vi "Setup.vi"(8 "error in (no error)":errorcluster, 10 "Setup Setting":T1 {"Interface:CAN:Termination" items=["Off", "On"]}, 11 "PXI 8513 in":refnum<class "PXI 8513.lvclass">) -> (0 "error out":errorcluster, 3 "PXI 8513 out":refnum<class "PXI 8513.lvclass">)   [LabVIEW 2023, in "CAN.lvlib" / "PXI 8513.lvclass"]
uses:
  PXI 8513.lvclass
  PXI 8513.lvclass/PXI 8513.ctl
  <resource>/objmgr/xnet.rc
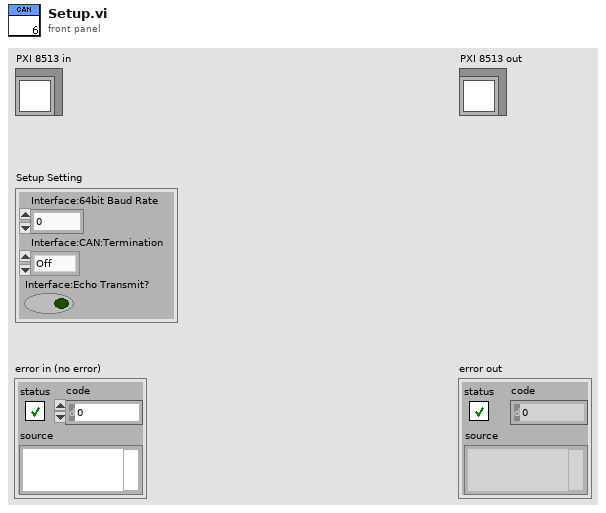
[diagram p1: front panel]
types:
  T1 = cluster{"Interface:64bit Baud Rate":u64, "Interface:CAN:Termination":u32, "Interface:Echo Transmit?":bool}
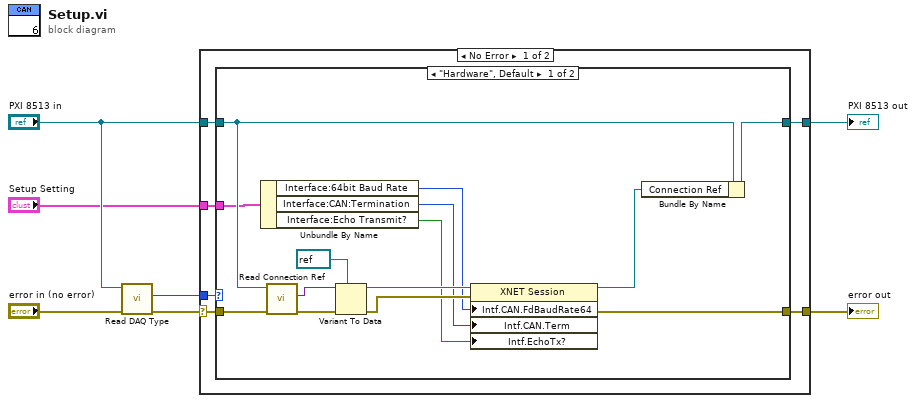
[diagram p0: block diagram]
diagram:
  n1 = call-dynamic "Read DAQ Type.vi"("error in (no error)"="error in (no error)", "PXI 8513 in"="PXI 8513 in") -> ("error out"=w6:errorcluster, "DAQ Type"=w5:enum16{"Hardware", "Simulation"})  [unwired: 7 in, 1 out]
  n2 = case shown="No Error" w6 {
    selector: w6 -> [w11 w30]
    tunnel: w5 -> [w13 _]
    tunnel: "PXI 8513 in" -> [w12 w31]
    tunnel: [w10 w31] -> w3
    tunnel: [w9 w30] -> w2
    tunnel: "Setup Setting" -> [w8 _]
    frame No Error {
      n3 = case shown="\"Hardware\", Default" w13 {
        tunnel: w12 -> [w22 w29]
        tunnel: w11 -> [w27 w28]
        tunnel: [w20 w29] -> w10
        tunnel: [w18 w28] -> w9
        tunnel: w8 -> [w17 _]
        frame "Hardware", Default {
          n4 = Unbundle By Name(w17) -> ("Interface:64bit Baud Rate"=w16:u64, "Interface:CAN:Termination"=w15:u32, "Interface:Echo Transmit?"=w14:bool)
          n5 = call-dynamic "Read Connection Ref.vi"("error in (no error)"=w27, "PXI 8513 in"=w22) -> ("error out"=w26:errorcluster, "Connection Ref"=w25:variant)  [unwired: 7 in, 1 out]
          n6 = Variant To Data(error in=w26, type=refnum<k21> refnum ("session out"), Variant=w25) -> (data=w23:refnum<k21>, error out=w21:errorcluster)
          n7 = property class="XNET Session"(reference=w23, error in=w21, "Intf.CAN.FdBaudRate64"=w16, "Intf.CAN.Term"=w15, "Intf.EchoTx?"=w14) -> (reference out=w19:refnum<k21>, error out=w18:errorcluster)
          n8 = Bundle By Name(cluster=w22, "Connection Ref"=w19) -> (w20:refnum<class "PXI 8513.lvclass">)
        }
        frame "Simulation" {
        }
      }
    }
    frame Error {
    }
  }
  "error out" <- w2
  "PXI 8513 out" <- w3
